vi "Test LabVIEW Build.vi"() -> ()   [LabVIEW 2014]
uses:
  Core/LabVIEW CI Service/Controls/Job Results - STYP.ctl
  Core/Shared/Controls/LabVIEW Build - STYP.ctl
  Core/LabVIEW CI Service/Classes/Job/Job.lvclass/Job.ctl
  Core/LabVIEW CI Service/Extensions/LabVIEW Build/LabVIEW Build/LabVIEW Build.lvclass
  Core/LabVIEW CI Service/Classes/Job/Job.lvclass
panel:
  out "error out":errorcluster
  out "Results":T1 {"Status" items=["Service Error"=504, "Abort"=503, "Fail"=500, "Pass"=200]}
  in  "LabVIEW Build":T2={"Executor_Number"="1", "Workspace_Path"=path "P:/alsmith/Sales/users/ACS/LabVIEW Continuous Integration/Workspace", "Build_Spec"="Cooler Executable", "Project_Path"=path "P:/alsmith/Sales/users/ACS/LabVIEW Continuous Integration/Test Project/Complete Solution - Cooler.lvproj", "Auto_Version_Increment"=FALSE}
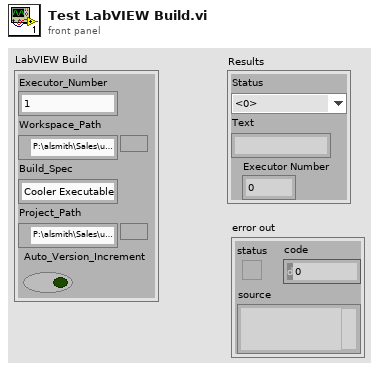
[diagram p1: front panel]
types:
  T1 = typedef "Job Results - STYP.ctl" = cluster{"Status":u16, "Text":string, "Executor Number":i32}
  T2 = cluster{"Executor_Number":string, "Workspace_Path":path, "Build_Spec":string, "Project_Path":path, "Auto_Version_Increment":bool}
  T3 = typedef "LabVIEW Build - STYP.ctl" = cluster{"Executor_Number":string, "Workspace_Path":string, "Build_Spec":string, "Target":string, "Project_Path":string, "Auto_Version_Increment":bool}
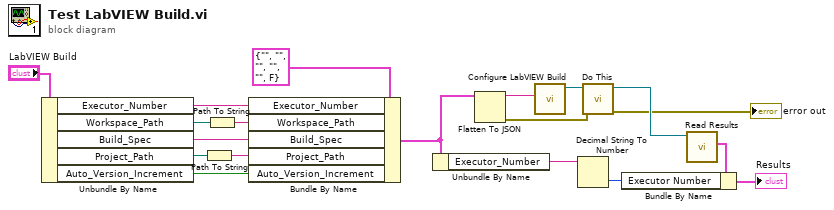
[diagram p0: block diagram]
diagram:
  n1 = Unbundle By Name("LabVIEW Build") -> ("Executor_Number"=w17:string, "Workspace_Path"=w13:path, "Build_Spec"=w15:string, "Project_Path"=w11:path, "Auto_Version_Increment"=w16:bool)
  n2 = Path To String(path=w11) -> (string=w10:string)
  n3 = Path To String(path=w13) -> (string=w12:string)
  n4 = Bundle By Name(cluster=T3 {"Executor_Number"="", "Workspace_Path"="", "Build_Spec"="", "Target"="", "Project_Path"="", "Auto_Version_Increment"=FALSE} ("LabVIEW Build"), "Executor_Number"=w17, "Workspace_Path"=w12, "Build_Spec"=w15, "Project_Path"=w10, "Auto_Version_Increment"=w16) -> (w8:T3)
  n5 = Unbundle By Name(w8) -> ("Executor_Number"=w19:string)
  n6 = Flatten To JSON(anything=w8) -> (JSON string=w7:string, 11:w5:errorcluster)  [unwired: 2 in]
  n7 = call "Configure LabVIEW Build.vi"("JSON string"=w7) -> ("EXE Build out"=w6:refnum<class "LabVIEW Build.lvclass">)  [unwired: 9 in, 1 out]
  n8 = Decimal String To Number(string=w19) -> (number=w9:i32)  [unwired: 2 in, 1 out]
  n9 = call-dynamic "Do This.vi"("error in (no error)"=w5, "LabVIEW Build in"=w6) -> ("error out"=→"error out":errorcluster, "LabVIEW Build out"=w4:refnum<class "LabVIEW Build.lvclass">)  [unwired: 8 in]
  n10 = call "Read Results.vi"("Job in"=w4) -> ("Results"=w3:T1)  [unwired: 10 in]
  n11 = Bundle By Name(cluster=w3, "Executor Number"=w9) -> (→"Results":T1)
